vi "Lab5, My auto save.vi"() -> ()   [LabVIEW 2010]
uses:
  <vilib>/Utility/file.llb/Write To Spreadsheet File (I64).vi
panel:
  out "Peak to Peak Diff":u16
  out "Previous Graph":u16[](graph)
  out "Current Graph":u16[](graph)
  in  "Data file path ending":string
  in  "time format string":string
  out "date/time string":string
  in  "AutoSave":bool
  out "Error Code":i32
  out "Error Message":string
  in  "InterChannel Delay":sgl=-1.0 format="%.2f"
  in  "Range":i32(ring)=1 items=["Not Programmable"=0, "+- 20 V"=27, "+- 10 V"=1, "+- 5 V"=2, "+- 4 V"=28, "+- 2.5 V"=3, "+- 2 V"=29, "+- 1.67 V"=4, "+- 1.25 V"=5, "+- 1 V"=6, "+- .625 V"=7, "+- .5 V"=8, "+- .25 V"=30, "+- .2 V"=31, "+- .1 V"=9, "+- .05 V"=10, "+- .01 V"=11, "+- .005 V"=12, "0 - 10 V"=13, "0 - 5 V"=14, "0 - 4 V"=36, "0 - 2.5 V"=15, "0 - 2 V"=16, "0 - 1.67 V"=17, "0 - 1.25 V"=18, "0 - 1 V"=19, "0 - .5 V"=32, "0 - .25 V"=33, "0 - .2 V"=34, "0 - .1 V"=20, "0 - .02 V"=35, "0 - .01 V"=21, "4 - 20 mA"=22, "2 - 10 mA"=23, "1 - 5 mA"=24, ".5 - 2.5 mA"=25, "0 - 20 mA"=26]
  in  "Options":i32
  in  "Rate":i32
  in  "Count":i32
  in  "Low Channel":i32
  in  "High Channel":i32
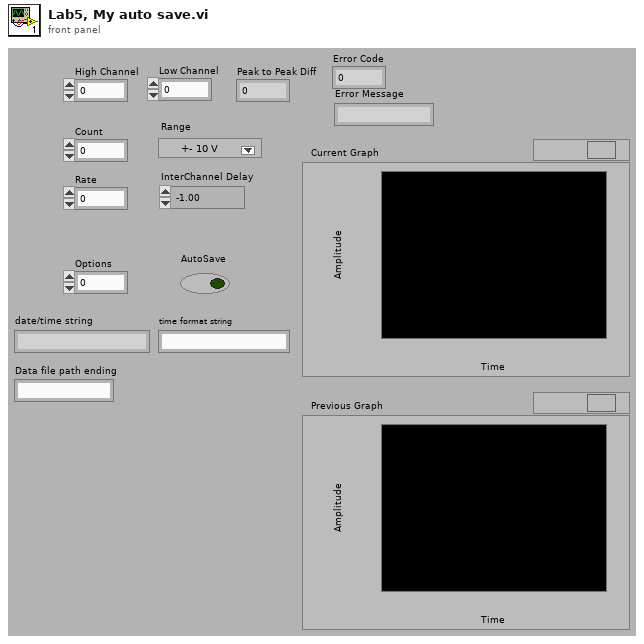
[diagram p1: front panel]
types:
  T1 = typedef "imagedata.ctl" = cluster{"image type":i32, "image depth":i32, "image":u8[], "mask":u8[], "colors":u32[], "Rectangle":cluster{"left":i16, "top":i16, "right":i16, "bottom":i16}}
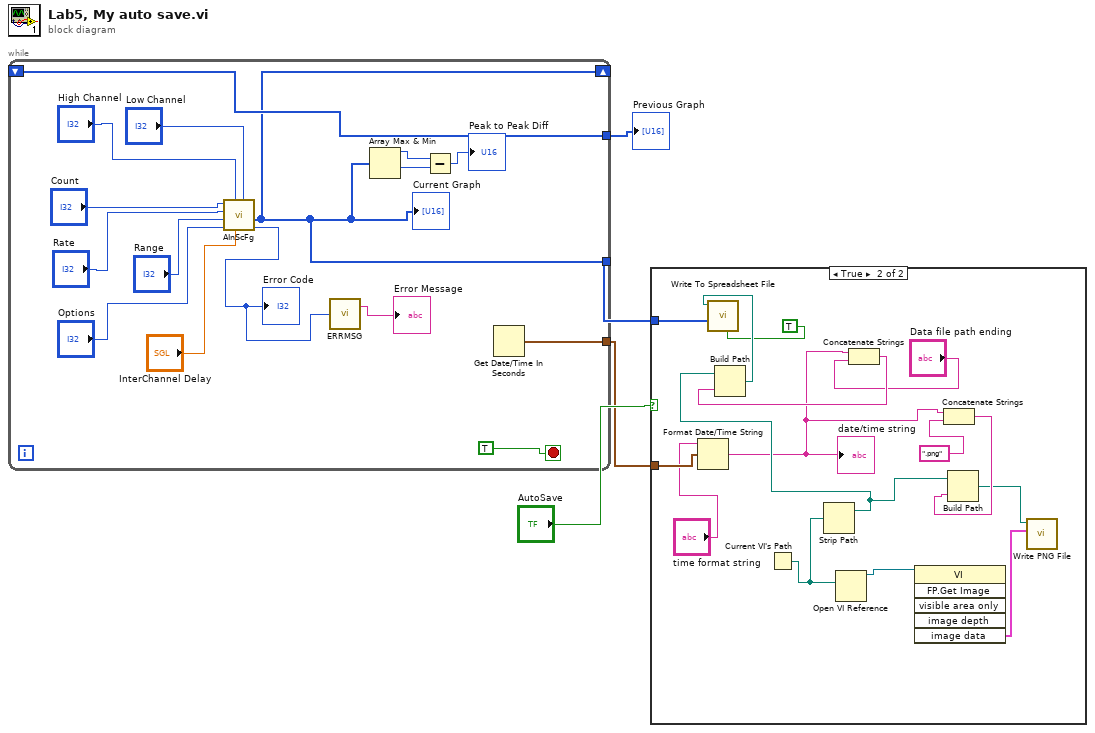
[diagram p0: block diagram]
diagram:
  n1 = while {
    shift-right: [w6] -> _
    shift-left: _ -> [w10]
    tunnel: [w10] -> w1
    tunnel: [w6] -> w3
    tunnel: [w9] -> w2
    stop <- TRUE stop-if-true
    n2 = call <menus>:"AInScFg.VI"("LowChan"="Low Channel", "InterChannel Delay"="InterChannel Delay", "HighChan"="High Channel", "Options"="Options", "Range"="Range", "Rate"="Rate", "Count"="Count") -> ("ErrCode"=w20:i32, "ADData"=w6:u16[])  [unwired: 1 in, 1 out]
    "Error Code" <- w20
    "Current Graph" <- w6
    n3 = call <menus>:"ERRMSG.VI"("ErrCode"=w20) -> ("ErrMsg"=→"Error Message":string)  [unwired: 1 out]
    n4 = Array Max & Min(array=w6) -> (max value=w7:u16, min value=w8:u16)  [unwired: 2 out]
    n5 = Subtract(x=w7, y=w8) -> (x-y=→"Peak to Peak Diff":u16)
    n6 = Get Date/Time In Seconds() -> (seconds since 1Jan1904=w9:timestamp)
  }
  "Previous Graph" <- w1
  n7 = case shown="True" "AutoSave" {
    tunnel: w3 -> [_ w35]
    tunnel: w2 -> [_ w32]
    frame False {
    }
    frame True {
      n8 = Format Date/Time String(time format string (%c)="time format string", seconds (now)=w32) -> (date/time string=w22:string)  [unwired: 1 in]
      "date/time string" <- w22
      n9 = Current VI's Path() -> (path=w26:path)
      n10 = Strip Path(path=w26) -> (stripped path=w27:path)  [unwired: 1 out]
      n11 = Open VI Reference(vi path=w26) -> (vi reference=w25:refnum<vi>)  [unwired: 5 in, 1 out]
      n12 = Concatenate Strings(w22, "Data file path ending") -> (w30:string)
      n13 = Build Path(base path=w27, name or relative path=w30) -> (appended path=w34:path)
      n14 = call-poly <vilib>:"Write To Spreadsheet File.vi"("transpose? (no:F)"=TRUE, "1D data"=w35, "file path (dialog if empty)"=w34) -> ()  [unwired: 5 in, 1 out]
      n15 = invoke class="VI" method="FP.Get Image"(reference=w25) -> ("image data"=w24:T1)  [unwired: 5 in, 5 out]
      n16 = Concatenate Strings(w22, ".png") -> (w28:string)
      n17 = Build Path(base path=w27, name or relative path=w28) -> (appended path=w23:path)
      n18 = call <vilib>:"Write PNG File.vi"("image data"=w24, "path to PNG file"=w23) -> ()  [unwired: 8 in, 2 out]
    }
  }
